vi "Update DMM Settings.vi"(2 "error in":errorcluster, 3 "DMM Measurement Type":i32(ring) items=["DC Volts", "AC Volts", "DC Current", "AC Current", "2-Wire Resistance", "Frequency", "Temperature", "Capacitance", "Continuity", "Diode", "4-Wire Resistance", "2nd DC Volts", "2nd AC Volts", "2nd DC Current", "2nd AC Current", "2nd Frequency"], 4 "DMM Model":T1, 5 "DMM Address":refnum<visa-resource-name>="GPIB0::5::INSTR") -> (0 "error out":errorcluster, 1 "VISA resource name out":refnum<visa-resource-name>)   [LabVIEW 2020]
uses:
  Typedefs/DMM Models Control.ctl
  <instrlib>/Agilent 34405/Agilent 34405.lvlib
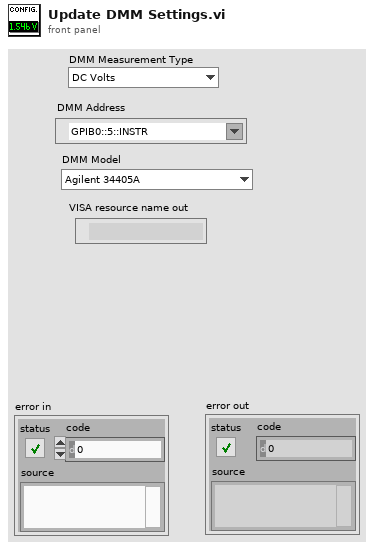
[diagram p1: front panel]
types:
  T1 = typedef "DMM Models Control.ctl" = enum16{"Agilent 34405A"}
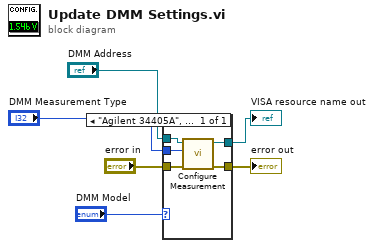
[diagram p0: block diagram]
diagram:
  n1 = case shown="\"Agilent 34405A\", Default" "DMM Model" {
    tunnel: "DMM Address" -> [w10]
    tunnel: "error in" -> [w9]
    tunnel: "DMM Measurement Type" -> [w11]
    tunnel: [w8] -> w2
    tunnel: [w7] -> w1
    frame "Agilent 34405A", Default {
      n2 = call <instrlib>:"Configure Measurement.vi"("error in (no error)"=w9, "Function (0: DC Volts)"=w11, "VISA resource name"=w10) -> ("error out"=w8:errorcluster, "VISA resource name out"=w7:refnum<visa-resource-name>)  [unwired: 7 in]
    }
  }
  "error out" <- w2
  "VISA resource name out" <- w1
